vi "Stepper Control DAQmx - 2009.vi"() -> ()   [LabVIEW 2009]
uses:
  <vilib>/DAQmx/create/channels.llb/DAQmx Create Channel (DO-Digital Output).vi
  <vilib>/Utility/error.llb/DialogType.ctl
  <vilib>/DAQmx/write.llb/DAQmx Write (Digital Bool 1Line 1Point).vi
panel:
  in  "High Time (ms)":u32
  in  "Low Time (ms)":u32
  in  "Position:":i16(knob)
  in  "Direction Control Output":tag caption="Direction Control Line:"
  in  "stop":bool
  in  "Pulse Output":tag caption="Stepper Output Line:"
  # "Pulse Characteristics:"
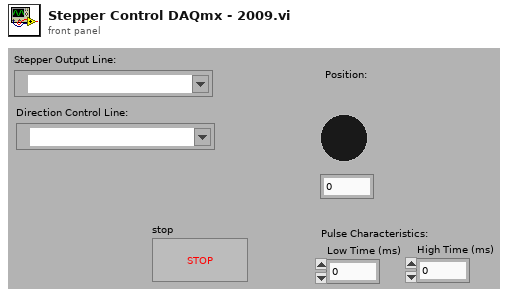
[diagram p1: front panel]
types:
  T1 = typedef "DialogType.ctl" = u16
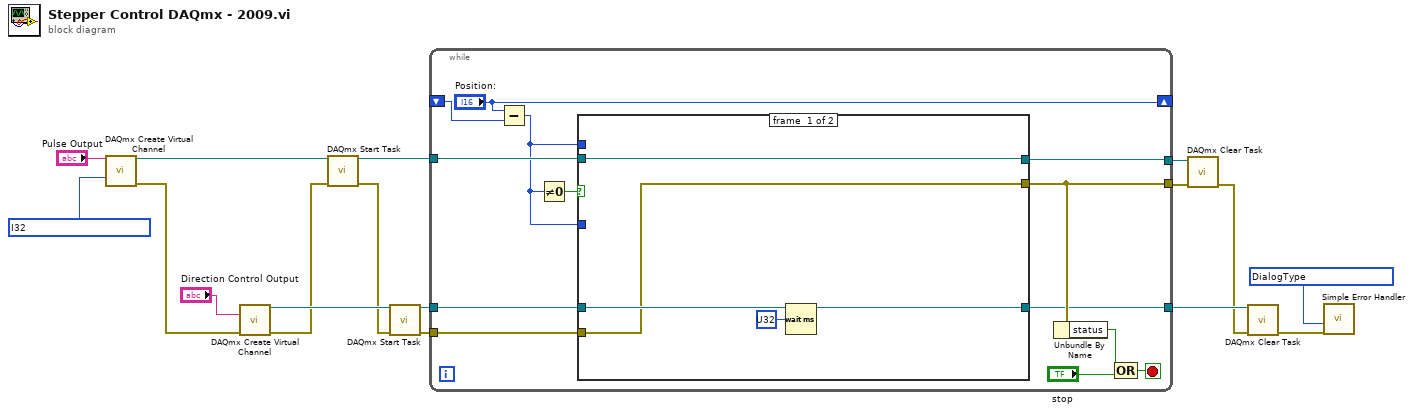
[diagram p0: block diagram]
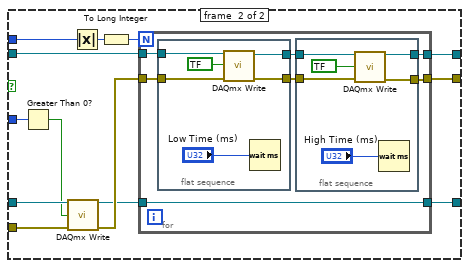
[diagram p2: hidden frame]
diagram:
  w14 = i32 ? items=["one channel for each line", "one channel for all lines"] ("line grouping")
  w16 = T1 ? items=["no dialog", "OK message", "continue or stop message", "OK message + warnings", "continue/stop + warnings"] ("type of dialog (OK msg:1)")
  n1 = call-poly <vilib>:"DAQmx Create Virtual Channel.vi"("lines"="Pulse Output", "line grouping"=w14) -> ("task out"=w13:refnum<k21>, "error out"=w6:errorcluster)  [unwired: 3 in, 9 out]
  n2 = call-poly <vilib>:"DAQmx Create Virtual Channel.vi"("lines"="Direction Control Output", "error in"=w6) -> ("task out"=w11:refnum<k21>, "error out"=w5:errorcluster)  [unwired: 3 in, 9 out]
  n3 = call <vilib>:"DAQmx Start Task.vi"("task/channels in"=w13, "error in"=w5) -> ("task out"=w12:refnum<k21>, "error out"=w4:errorcluster)  [unwired: 12 out]
  n4 = call <vilib>:"DAQmx Start Task.vi"("task/channels in"=w11, "error in"=w4) -> ("task out"=w10:refnum<k21>, "error out"=w9:errorcluster)  [unwired: 12 out]
  n5 = while {
    shift-right: ["Position:"] -> _
    shift-left: _ -> [w30]
    tunnel: w12 -> [w28]
    tunnel: w10 -> [w27]
    tunnel: w9 -> [w26]
    tunnel: [w25] -> w7
    tunnel: [w24] -> w8
    tunnel: [w20] -> w3
    stop <- w21 stop-if-true
    n6 = Subtract(x="Position:", y=w30) -> (x-y=w18:i16)
    n7 = Not Equal To 0?(x=w18) -> (x != 0?=w19:bool)
    n8 = case shown="True" w19 {
      tunnel: w28 -> [w33 w47]
      tunnel: w27 -> [w34 w46]
      tunnel: w26 -> [w31 w45]
      tunnel: [w33 w43] -> w25
      tunnel: [w31 w41] -> w24
      tunnel: [w34 w40] -> w20
      tunnel: w18 -> [_ w38]
      tunnel: w18 -> [_ w35]
      frame #0 {
        n9 = Wait (ms)(milliseconds to wait=u32 ?) -> ()  [unwired: 1 out]
      }
      frame #1 {
        n10 = Greater Than 0?(x=w38) -> (x > 0?=w39:bool)
        n11 = call-poly <vilib>:"DAQmx Write.vi"("task/channels in"=w46, "data"=w39, "error in"=w45) -> ("task out"=w42:refnum<k21>, "error out"=w44:errorcluster)  [unwired: 1 in, 10 out]
        n12 = Absolute Value(x=w35) -> (abs(x)=w37:i16)
        n13 = To Long Integer(number=w37) -> (32bit integer=w36:i32)
        n14 = for {
          N: w36 -> [_]
          tunnel: w47 -> [w54]
          tunnel: w44 -> [w53]
          tunnel: [w51] -> w43
          tunnel: [w49] -> w41
          tunnel: w42 -> [w50]
          tunnel: [w50] -> w40
          n15 = flat-sequence {
            tunnel: w54 -> [w66]
            tunnel: w53 -> [w65]
            tunnel: [w64] -> w52
            tunnel: [w62] -> w48
            frame #0 {
              n16 = call-poly <vilib>:"DAQmx Write.vi"("task/channels in"=w66, "data"=bool ?, "error in"=w65) -> ("task out"=w64:refnum<k21>, "error out"=w62:errorcluster)  [unwired: 1 in, 10 out]
              n17 = Wait (ms)(milliseconds to wait="Low Time (ms)") -> ()  [unwired: 1 out]
            }
          }
          n18 = flat-sequence {
            tunnel: w52 -> [w60]
            tunnel: [w59] -> w51
            tunnel: [w57] -> w49
            tunnel: w48 -> [w56]
            frame #0 {
              n19 = call-poly <vilib>:"DAQmx Write.vi"("task/channels in"=w60, "data"=bool ?, "error in"=w56) -> ("task out"=w59:refnum<k21>, "error out"=w57:errorcluster)  [unwired: 1 in, 10 out]
              n20 = Wait (ms)(milliseconds to wait="High Time (ms)") -> ()  [unwired: 1 out]
            }
          }
        }
      }
    }
    n21 = Unbundle By Name(w24) -> ("status"=w22:bool)
    n22 = Compound Arithmetic op=OR(w22, "stop") -> (w21:bool)
  }
  n23 = call <vilib>:"DAQmx Clear Task.vi"("task in"=w7, "error in"=w8) -> ("error out"=w2:errorcluster)  [unwired: 13 out]
  n24 = call <vilib>:"DAQmx Clear Task.vi"("task in"=w3, "error in"=w2) -> ("error out"=w1:errorcluster)  [unwired: 13 out]
  n25 = call <vilib>:"Simple Error Handler.vi"("type of dialog (OK msg:1)"=w16, "error in (no error)"=w1) -> ()  [unwired: 8 out]
